vi "Get Setting.vi"(0 "Setting name":string, 11 "error in (no error)":errorcluster) -> (4 "Setting value out":string, 6 "Setting empty or not found?":bool, 15 "error out":errorcluster)   [LabVIEW 2023, in "RFCalAndFixtureCharact.Common.lvlib"]
uses:
  RFCalAndFixtureCharact.Common.lvlib
  Type Definitions/Dictionary Operation.ctl
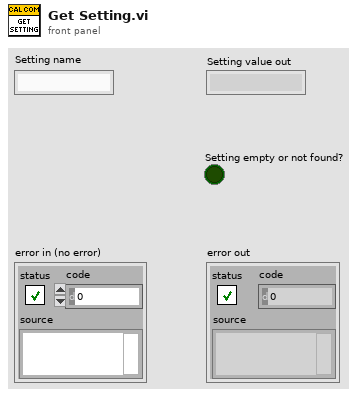
[diagram p1: front panel]
types:
  T1 = typedef "RFCalAndFixtureCharact.Common.lvlib/Dictionary Operation.ctl" = enum16{"Read", "Insert", "Remove", "Clear", "Get All", "Update"}
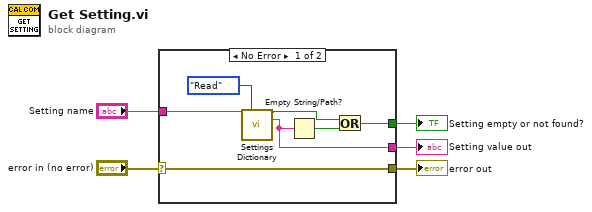
[diagram p0: block diagram]
diagram:
  n1 = case shown="No Error" "error in (no error)" {
    selector: "error in (no error)" -> [w12 w13]
    tunnel: "Setting name" -> [w10 _]
    tunnel: [w9 _] -> w4
    tunnel: [w12 w13] -> w2
    tunnel: [w6 _] -> w1
    frame No Error {
      n2 = call "Settings Dictionary.vi"("Setting name"=w10, "Action"=Dictionary_Operation."Read") -> ("Setting already included? / Setting not found?"=w7:bool, "Setting value out"=w9:string)  [unwired: 12 in]
      n3 = Empty String/Path?(string/path=w9) -> (empty?=w8:bool)
      n4 = Or(x=w7, y=w8) -> (x .or. y?=w6:bool)
    }
    frame Error {
    }
  }
  "error out" <- w2
  "Setting value out" <- w4
  "Setting empty or not found?" <- w1
